vi "SortByClassName.vi"(1 "Children In Memory":refnum<vi>[](array[refnum])) -> (0 "Sorted Array":refnum<vi>[](array[refnum]))   [LabVIEW 2017, in "DynamicDispatchImplementationWalker.lvlib"]
uses:
  DynamicDispatchImplementationWalker.lvlib
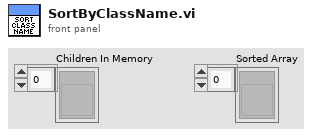
[diagram p1: front panel]
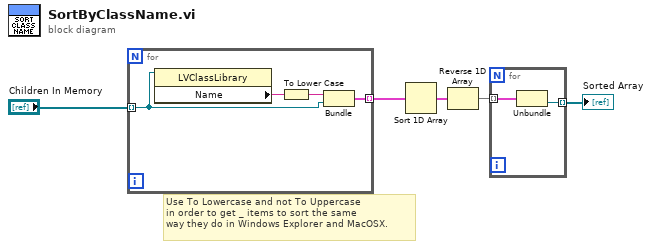
[diagram p0: block diagram]
diagram:
  # "Use To Lowercase and not To Uppercase\nin order to get _ items to sort the same\nway they do in Windows Explorer and MacOSX."
  n1 = for {
    tunnel: "Children In Memory" -> [w8] mode=indexing
    tunnel: [w7] -> w1 mode=indexing
    n2 = property class="LVClassLibrary"(reference=w8) -> ("Name"=w9:string)  [unwired: 1 in, 2 out]
    n3 = To Lower Case(string=w9) -> (all lower case string=w6:string)
    n4 = Bundle(w6, w8) -> (w7:cluster{string, refnum<vi>})  [unwired: 1 in]
  }
  n5 = Sort 1D Array(array=w1) -> (sorted array=w2:cluster{string, refnum<vi>}[])
  n6 = Reverse 1D Array(array=w2) -> (reversed array=w5:cluster{string, refnum<vi>}[])
  n7 = for {
    tunnel: w5 -> [w11] mode=indexing
    tunnel: [w10] -> w4 mode=indexing
    n8 = Unbundle(w11) -> (w10:refnum<vi>)  [unwired: 1 out]
  }
  "Sorted Array" <- w4
